vi "Get Model Parameters - from Model File.vi"(0 "Model Parameter Filepath (.txt)":path, 11 "Error (in)":errorcluster) -> (8 "Parameters":string[](array[string]), 15 "Error (out)":errorcluster)   [LabVIEW 2016, in "System Mapping Tool.lvlib"]
uses:
  <vilib>/Utility/file.llb/Read Delimited Spreadsheet (string).vi
  System Mapping Tool.lvlib
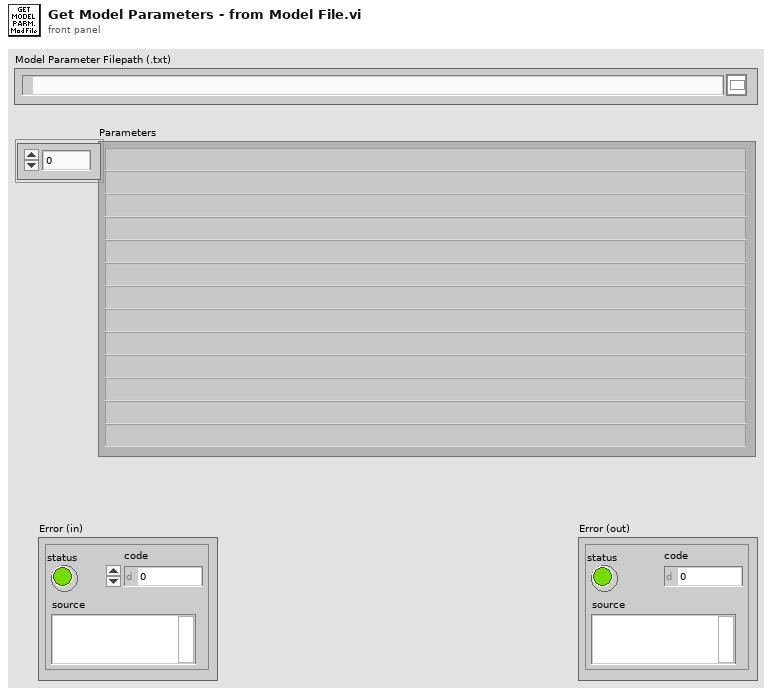
[diagram p1: front panel]
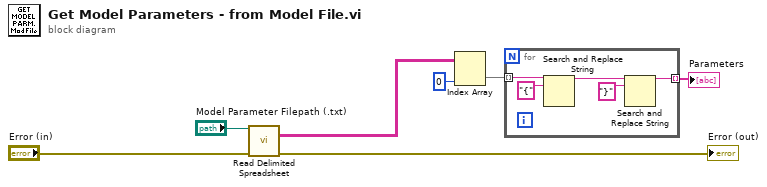
[diagram p0: block diagram]
diagram:
  n1 = call-poly <vilib>:"Read Delimited Spreadsheet.vi"("file path (dialog if empty)"="Model Parameter Filepath (.txt)", "error in (no error)"="Error (in)") -> ("all rows"=w6:string[][], "error out"=→"Error (out)":errorcluster)  [unwired: 8 in, 4 out]
  n2 = Index Array(array=w6, index (col)=0 ("disabled index (col)")) -> (element=w4:string[])  [unwired: 1 in]
  n3 = for {
    tunnel: w4 -> [w12] mode=indexing
    tunnel: [w8] -> w3 mode=indexing
    n4 = Search and Replace String(input string=w12, search string="{") -> (result string=w9:string)  [unwired: 6 in, 3 out]
    n5 = Search and Replace String(input string=w9, search string="}") -> (result string=w8:string)  [unwired: 6 in, 3 out]
  }
  "Parameters" <- w3
